vi "Update Trig Line.vi"(8 "error in (no error)":errorcluster, 9 "PB Trigger Line":i32, 10 "Triggering":bool[](array[boolean]), 11 "Pulseblaster in":refnum<class "Pulseblaster.lvclass">) -> (0 "error out":errorcluster, 3 "Pulseblaster out":refnum<class "Pulseblaster.lvclass">)   [LabVIEW 2013, in "Pulseblaster.lvclass"]
uses:
  Pulseblaster.lvclass
  Pulseblaster.lvclass/Pulseblaster.ctl
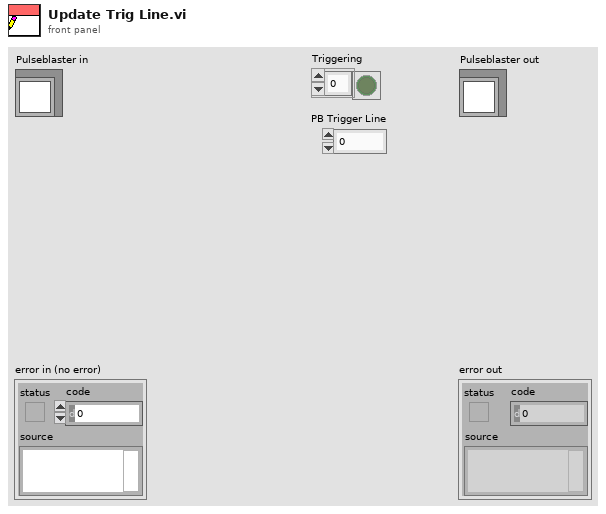
[diagram p1: front panel]
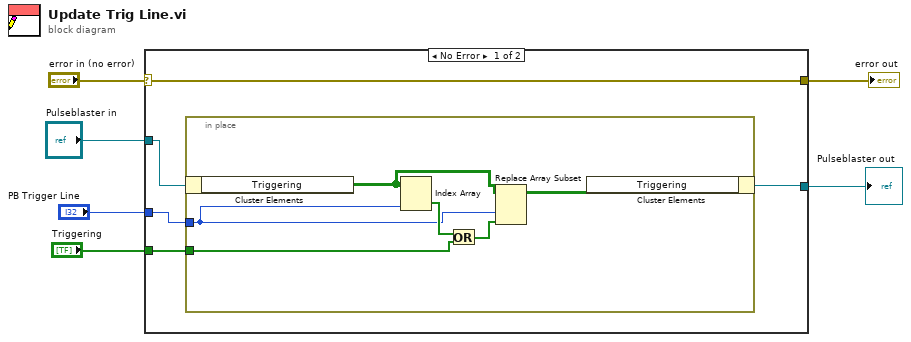
[diagram p0: block diagram]
diagram:
  n1 = case shown="No Error" "error in (no error)" {
    selector: "error in (no error)" -> [w11 w18]
    tunnel: [w11 w18] -> w5
    tunnel: [w7 w19] -> w4
    tunnel: "Pulseblaster in" -> [w10 w19]
    tunnel: "Triggering" -> [w9 _]
    tunnel: "PB Trigger Line" -> [w8 _]
    frame No Error {
      n2 = in-place {
        in-place-border: w9 -> [w16]
        in-place-border: w8 -> [w12]
        n3 = in-place-cluster #1(w10) -> ("Triggering"=w15:bool[][])
        n4 = Index Array(array=w15, index (col)=w12) -> (element=w17:bool[])  [unwired: 1 in]
        n5 = Or(x=w17, y=w16) -> (x .or. y?=w13:bool[])
        n6 = Replace Array Subset(array=w15, new element=w13, index (col)=w12) -> (w14:bool[][])  [unwired: 1 in]
        n7 = in-place-cluster #1("Triggering"=w14) -> (w7:refnum<class "Pulseblaster.lvclass">)
      }
    }
    frame Error {
    }
  }
  "error out" <- w5
  "Pulseblaster out" <- w4
